vi "Static Write.vi"(8 "error in (no error)":errorcluster, 10 "Value":cdb, 11 "Abs_Complex Double Float in":refnum<class "Abs_Complex Double Float.lvclass">) -> (0 "error out":errorcluster, 3 "Abs_Complex Double Float out":refnum<class "Abs_Complex Double Float.lvclass">)   [LabVIEW 2021, in "Abs_Complex Double Float.lvclass"]
uses:
  Abs_Complex Double Float.lvclass
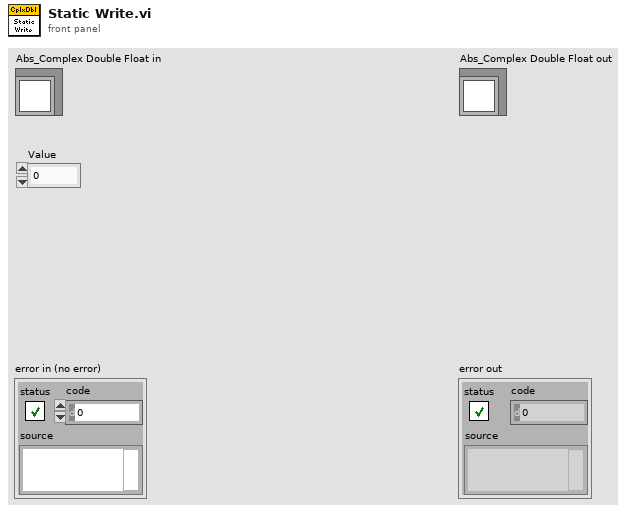
[diagram p1: front panel]
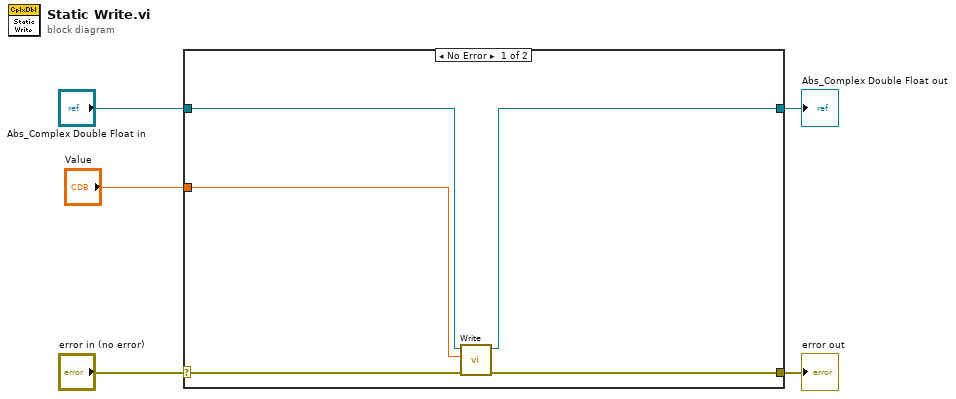
[diagram p0: block diagram]
diagram:
  n1 = case shown="No Error" "error in (no error)" {
    selector: "error in (no error)" -> [w10 w12]
    tunnel: [w9 w12] -> w4
    tunnel: [w7 w11] -> w2
    tunnel: "Abs_Complex Double Float in" -> [w8 w11]
    tunnel: "Value" -> [w6 _]
    frame No Error {
      n2 = call-dynamic "Write.vi"("error in (no error)"=w10, "Value"=w6, "Double Float.lvclass_340760 in"=w8) -> ("error out"=w9:errorcluster, "Double Float.lvclass_340760 out"=w7:refnum<class "Abs_Complex Double Float.lvclass">)  [unwired: 7 in]
    }
    frame Error {
    }
  }
  "error out" <- w4
  "Abs_Complex Double Float out" <- w2
